vi "Write Downscale Factor.vi"(8 "error in (no error)":errorcluster, 10 "Downscale Factor":u8, 11 "ZXing Options in":refnum<class "ZXing Options.lvclass">) -> (0 "error out":errorcluster, 3 "ZXing Options out":refnum<class "ZXing Options.lvclass">)   [LabVIEW 2020, in "feature_detection.lvlib" / "ZXing Options.lvclass"]
uses:
  ZXing Options.lvclass
  ZXing Options.lvclass/ZXing Options.ctl
  Field.ctl
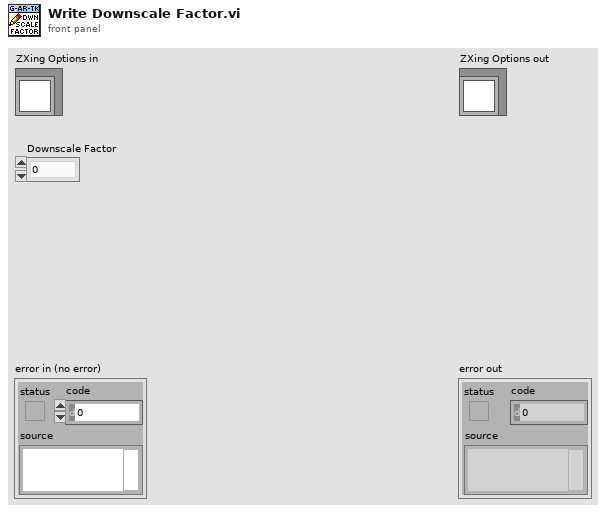
[diagram p1: front panel]
types:
  T1 = typedef "feature_detection.lvlib/ZXing Options.lvclass/Field.ctl" = enum8{"Try Harder", "Try Rotate", "Try Invert", "Try Downscale", "Is Pure", "Try Code 39 Ext Mode", "Return Errors", "Downscale Factor", "Min Line Count", "Max Number of Symbols", "Binarizer", "EAN Add On Symbol", "Text Mode", "Character Set", "Downscale Threshold"}
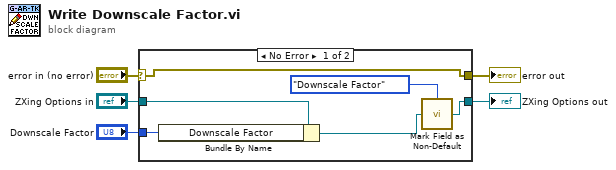
[diagram p0: block diagram]
diagram:
  n1 = case shown="No Error" "error in (no error)" {
    selector: "error in (no error)" -> [w11 w12]
    tunnel: [w11 w12] -> w4
    tunnel: [w7 w13] -> w2
    tunnel: "ZXing Options in" -> [w10 w13]
    tunnel: "Downscale Factor" -> [w8 _]
    frame No Error {
      n2 = Bundle By Name(cluster=w10, "Downscale Factor"=w8) -> (w9:refnum<class "ZXing Options.lvclass">)
      n3 = call "Mark Field as Non-Default.vi"("ZXing Options in"=w9, "Field"=Field."Downscale Factor") -> ("ZXing Options out"=w7:refnum<class "ZXing Options.lvclass">)
    }
    frame Error {
    }
  }
  "error out" <- w4
  "ZXing Options out" <- w2
